vi "Set Digital Out.vi"(0 "connection ID":refnum<k16>, 1 "address":u32, 2 "port":u16, 5 "IO State":T1 items=["LOW", "HIGH"], 9 "timeout ms (1000)":i32=1000, 11 "error in (no error)":errorcluster) -> (4 "connection ID out":refnum<k16>, 6 "received data":string, 8 "Relays":bool[](array[boolean]), 15 "error out":errorcluster)   [LabVIEW 2016]
uses:
  instr.lvlib
  IO State.ctl
panel:
  in  "IO Number":u16
  out "Send String":string
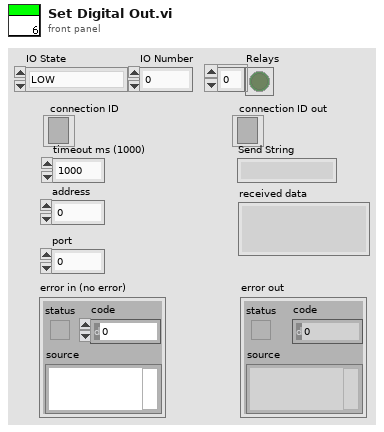
[diagram p1: front panel]
types:
  T1 = typedef "GSI-AF-IO.lvlib/Controllino Mega.lvlib/instr.lvlib/IO State.ctl" = u16
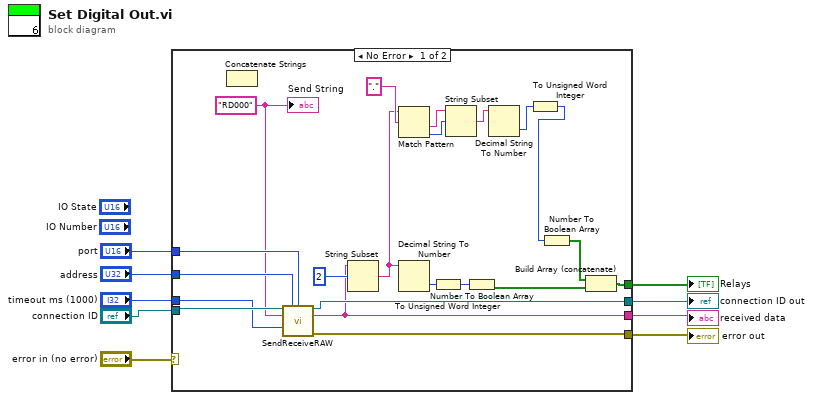
[diagram p0: block diagram]
diagram:
  n1 = case shown="No Error" "error in (no error)" {
    selector: "error in (no error)" -> [_ w32]
    tunnel: [w30 w32] -> w9
    tunnel: "timeout ms (1000)" -> [w27 _]
    tunnel: "connection ID" -> [w28 w31]
    tunnel: [w29 w31] -> w5
    tunnel: "address" -> [w26 _]
    tunnel: "port" -> [w25 _]
    tunnel: [w22 _] -> w2
    tunnel: [w16 _] -> w1
    frame No Error {
      w24 = "RD000" ("data in")
      n2 = Concatenate Strings() -> ()  [unwired: 2 in, 1 out]
      n3 = call "SendReceiveRAW.vi"("connection ID"=w28, "address"=w26, "port"=w25, "RAW data in"=w24, "timeout ms (1000)"=w27) -> ("connection ID out"=w29:refnum<k16>, "received data"=w22:string, "error out"=w30:errorcluster)  [unwired: 8 in]
      n4 = String Subset(string=w22, offset (0)=2 ("offset")) -> (substring=w20:string)  [unwired: 1 in]
      n5 = Match Pattern(string=w20, regular expression=".") -> (after substring=w18:string, offset past match=w19:i32)  [unwired: 1 in, 2 out]
      n6 = Decimal String To Number(string=w20) -> (number=w14:i32)  [unwired: 2 in, 1 out]
      n7 = To Unsigned Word Integer(number=w14) -> (unsigned 16bit integer=w15:u16)
      n8 = String Subset(string=w18, offset (0)=w19) -> (substring=w17:string)  [unwired: 1 in]
      n9 = Number To Boolean Array(number=w15) -> (Boolean array=w10:bool[])
      n10 = Decimal String To Number(string=w17) -> (number=w13:i32)  [unwired: 2 in, 1 out]
      n11 = To Unsigned Word Integer(number=w13) -> (unsigned 16bit integer=w12:u16)
      n12 = Number To Boolean Array(number=w12) -> (Boolean array=w11:bool[])
      n13 = Build Array (concatenate)(w11, w10) -> (w16:bool[])
      "Send String" <- w24
    }
    frame Error {
    }
  }
  "error out" <- w9
  "received data" <- w2
  "connection ID out" <- w5
  "Relays" <- w1
